vi "CPU Load Benchmark.vi"(8 "error in (no error)":errorcluster, 11 "SV B-M (Host) in":refnum<class "SV B-M (Host).lvclass">) -> (0 "error out":errorcluster, 3 "SV B-M (Host) out":refnum<class "SV B-M (Host).lvclass">)   [LabVIEW 2015, in "SV B-M (Host).lvclass"]
doc: "Open connections to all the shared variables that were deployed. Send a command to the target to do the same and wait for acknowledgement that was completed."
uses:
  SV B-M (Host).lvclass
  SV B-M (Host).lvclass/SV B-M (Host).ctl
  Listbox - In Progress.vi
  Command & Ack - Send Command.vi
  Command & Ack - Receive Ack.vi
  Process Ack Data - CPU Load BM.vi
  Listbox - Complete.vi
panel:
  out "SV Data":variant[][](array[variant])
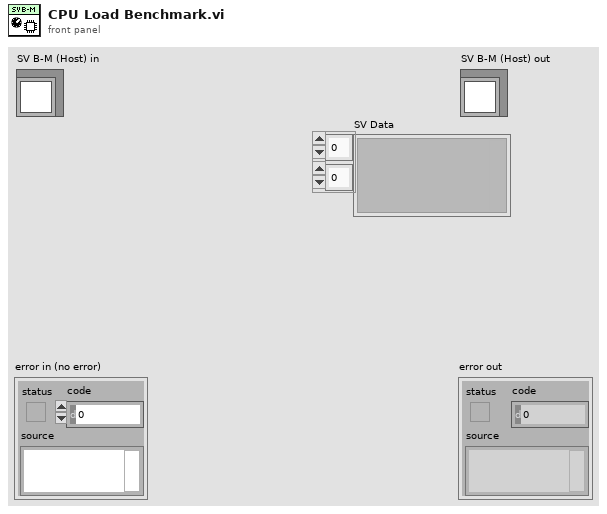
[diagram p1: front panel]
types:
  T1 = typedef "Variable Data Type.ctl" = enum16{"U8", "U16", "U32", "U64", "I8", "I16", "I32", "I64", "Single", "Double", "Boolean", "String"}
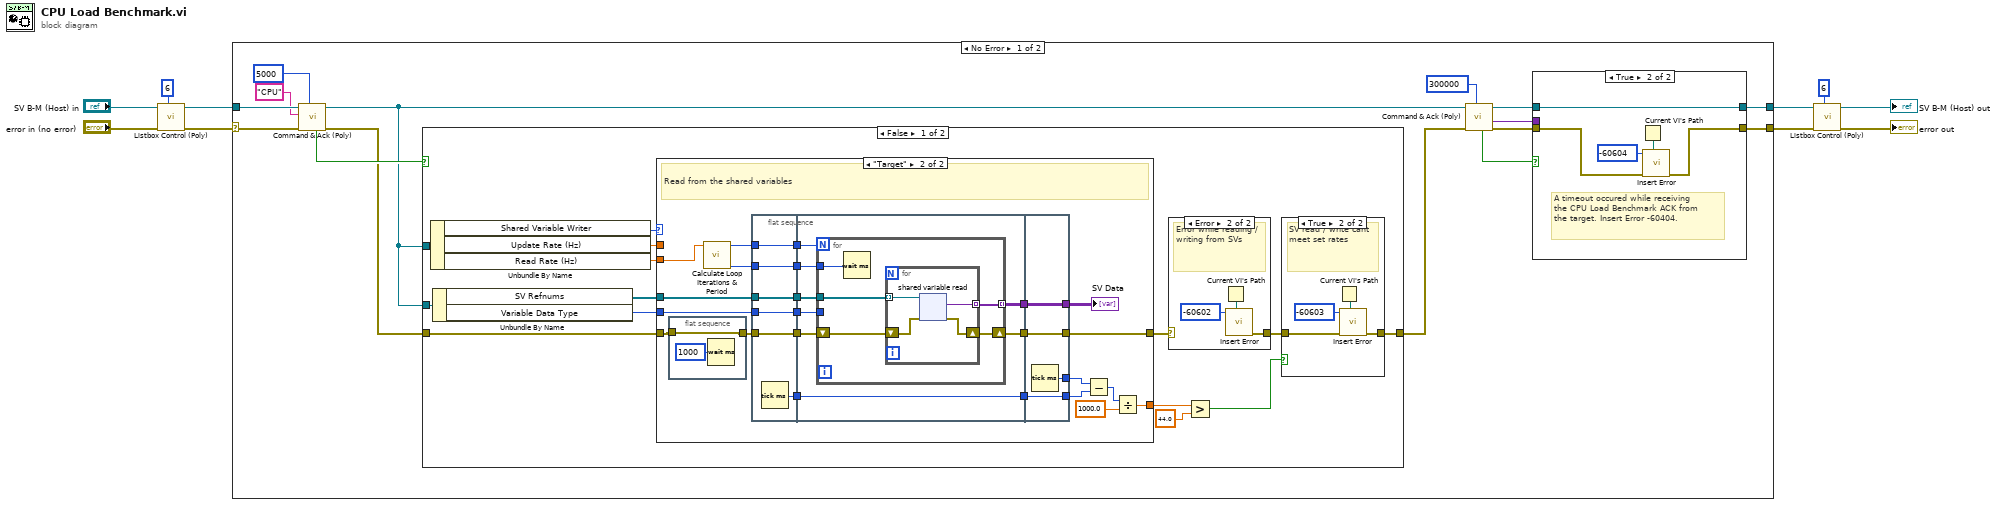
[diagram p0: block diagram]
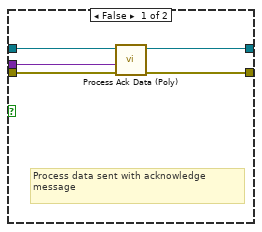
[diagram p2: hidden frame]
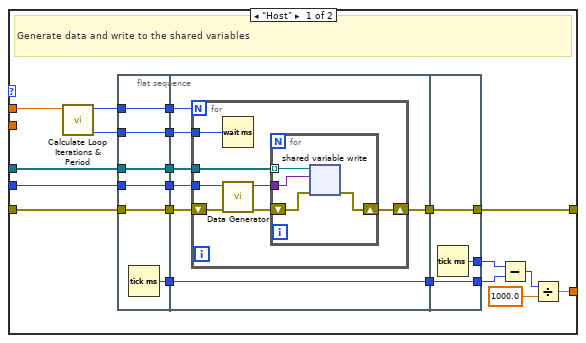
[diagram p5: hidden frame]
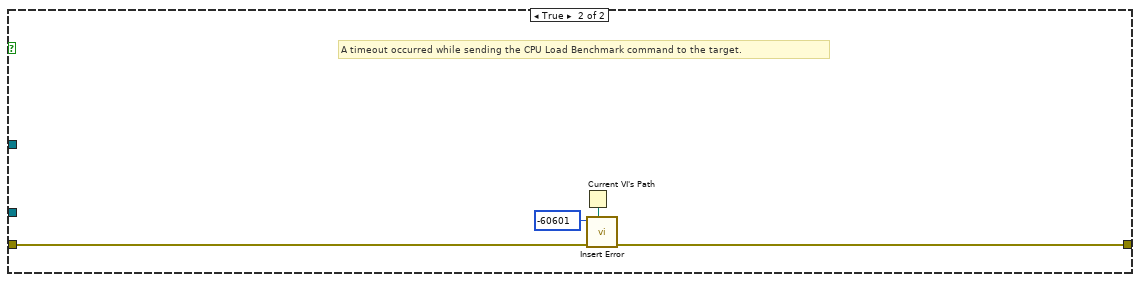
[diagram p6: hidden frame]
diagram:
  n1 = call-poly "Listbox Control (Poly).vi"("Row to Update"=6, "error in (no error)"="error in (no error)", "SV B-M In"="SV B-M (Host) in") -> ("error out"=w7:errorcluster, "SV B-M Out"=w8:refnum<class "SV B-M (Host).lvclass">)  [unwired: 7 in]
  n2 = case shown="No Error" w7 {
    selector: w7 -> [w24 w163]
    tunnel: [w12 w163] -> w3
    tunnel: [w13 w162] -> w4
    tunnel: w8 -> [w25 w162]
    frame No Error {
      n3 = call-poly "Command & Ack (Poly).vi"("Timeout (-1)"=5000, "error in (no error)"=w24, "Message"="CPU", "SV B-M (Host) in"=w25) -> ("error out"=w19:errorcluster, "SV B-M (Host) out"=w18:refnum<class "SV B-M (Host).lvclass">, "Timeout?"=w20:bool)  [unwired: 5 in]
      n4 = case shown="False" w20 {
        tunnel: w19 -> [w42 w161]
        tunnel: w18 -> [w49 _]
        tunnel: w18 -> [w45 _]
        tunnel: [w36 w158] -> w17
        frame False {
          n5 = Unbundle By Name(w49) -> ("Shared Variable Writer"=w48:enum16{"Target", "Host"}, "Update Rate (Hz)"=w47:dbl, "Read Rate (Hz)"=w46:dbl)
          n6 = Unbundle By Name(w45) -> ("SV Refnums"=w44:refnum<k21>[], "Variable Data Type"=w43:T1)
          n7 = case shown="\"Target\"" w48 {
            tunnel: w47 -> [w78 _]
            tunnel: w46 -> [_ w111]
            tunnel: w44 -> [w75 w126]
            tunnel: w43 -> [w74 w125]
            tunnel: w42 -> [w69 w107]
            tunnel: [w60 w112] -> w41
            tunnel: [w59 w109] -> w39
            frame "Host" {
              # "Generate data and write to the shared variables"
              n8 = call "Calculate Loop Iterations & Period.vi"("Rate"=w78) -> ("Wait (ms)"=w76:u32, "# Iterations"=w77:i32)  [unwired: 9 in]
              n9 = flat-sequence {
                tunnel: w74 -> [w81]
                tunnel: w75 -> [w82]
                tunnel: w76 -> [w83]
                tunnel: w77 -> [w84]
                tunnel: [w84] -> w73
                tunnel: [w83] -> w72
                tunnel: [w82] -> w71
                tunnel: [w81] -> w70
                tunnel: w69 -> [w80]
                tunnel: [w80] -> w68
                tunnel: [w79] -> w67
                tunnel: w73 -> [w91]
                tunnel: w72 -> [w90]
                tunnel: w71 -> [w89]
                tunnel: w70 -> [w88]
                tunnel: w68 -> [w87]
                tunnel: w67 -> [w86]
                tunnel: [w86] -> w66
                tunnel: [w85] -> w65
                tunnel: [w105] -> w64
                tunnel: w66 -> [w105]
                tunnel: w65 -> [w103]
                tunnel: [w104] -> w63
                tunnel: [w103] -> w59
                frame #0 {
                  n10 = Tick Count (ms)() -> (millisecond timer value=w79:u32)
                }
                frame #1 {
                  n11 = for {
                    N: w91 -> [_]
                    tunnel: w90 -> [w98]
                    tunnel: w89 -> [w95]
                    tunnel: w88 -> [w97]
                    shift-right: [w92] -> w85
                    shift-left: w87 -> [w96]
                    n12 = Wait (ms)(milliseconds to wait=w98) -> ()  [unwired: 1 out]
                    n13 = call "Data Generator.vi"("error in (no error)"=w96, "Variable Data Type"=w97) -> ("error out"=w93:errorcluster, "Variant"=w94:variant)  [unwired: 8 in]
                    n14 = for {
                      tunnel: w95 -> [w102] mode=indexing
                      tunnel: w94 -> [w100]
                      shift-right: [w99] -> w92
                      shift-left: w93 -> [w101]
                      n15 = shared-variable-write(w102, w101, w100) -> (w99:errorcluster)  [unwired: 1 out]
                    }
                  }
                }
                frame #2 {
                  n16 = Tick Count (ms)() -> (millisecond timer value=w104:u32)
                }
              }
              n17 = Subtract(x=w63, y=w64) -> (x-y=w62:u32)
              n18 = Divide(x=w62, y=1000.0) -> (x/y=w60:dbl)
            }
            frame "Target" {
              # "Read from the shared variables"
              n19 = flat-sequence {
                tunnel: [w130] -> w106
                tunnel: w107 -> [w130]
                frame #0 {
                  n20 = Wait (ms)(milliseconds to wait=u32 1000) -> ()  [unwired: 1 out]
                }
              }
              n21 = call "Calculate Loop Iterations & Period.vi"("Rate"=w111) -> ("Wait (ms)"=w127:u32, "# Iterations"=w128:i32)  [unwired: 9 in]
              n22 = flat-sequence {
                tunnel: w125 -> [w133]
                tunnel: w126 -> [w134]
                tunnel: w127 -> [w135]
                tunnel: w128 -> [w136]
                tunnel: [w136] -> w124
                tunnel: [w135] -> w123
                tunnel: [w134] -> w122
                tunnel: [w133] -> w121
                tunnel: w106 -> [w132]
                tunnel: [w132] -> w120
                tunnel: [w131] -> w119
                tunnel: w124 -> [w144]
                tunnel: w123 -> [w143]
                tunnel: w122 -> [w142]
                tunnel: w121 -> [w141]
                tunnel: w120 -> [w140]
                tunnel: w119 -> [w139]
                tunnel: [w139] -> w118
                tunnel: [w138] -> w117
                tunnel: [w137] -> w110
                tunnel: [w157] -> w116
                tunnel: w118 -> [w157]
                tunnel: w117 -> [w154]
                tunnel: [w156] -> w115
                tunnel: [w155] -> w108
                tunnel: w110 -> [w155]
                tunnel: [w154] -> w109
                frame #0 {
                  n23 = Tick Count (ms)() -> (millisecond timer value=w131:u32)
                }
                frame #1 {
                  n24 = for {
                    N: w144 -> [_]
                    tunnel: w143 -> [w149]
                    tunnel: w142 -> [w148]
                    tunnel: w141 -> [_]
                    shift-right: [w147] -> w138
                    shift-left: w140 -> [w146]
                    tunnel: [w145] -> w137 mode=indexing
                    n25 = Wait (ms)(milliseconds to wait=w149) -> ()  [unwired: 1 out]
                    n26 = for {
                      tunnel: w148 -> [w153] mode=indexing
                      shift-right: [w151] -> w147
                      shift-left: w146 -> [w152]
                      tunnel: [w150] -> w145 mode=indexing
                      n27 = shared-variable-read(w153, w152) -> (w151:errorcluster, w150:variant)  [unwired: 2 out]
                    }
                  }
                }
                frame #2 {
                  n28 = Tick Count (ms)() -> (millisecond timer value=w156:u32)
                }
              }
              n29 = Subtract(x=w115, y=w116) -> (x-y=w114:u32)
              n30 = Divide(x=w114, y=1000.0) -> (x/y=w112:dbl)
              "SV Data" <- w108
            }
          }
          n31 = case shown="Error" w39 {
            selector: w39 -> [w55 _]
            tunnel: [w55 w56] -> w38
            frame No Error {
              # "No Error"
            }
            frame Error {
              # "Error while reading / writing from SVs"
              n32 = Current VI's Path() -> (path=w58:path)
              n33 = call "Insert Error.vi"("VI Path"=w58, "Error Code"=-60602) -> ("error out"=w56:errorcluster)  [unwired: 9 in]
            }
          }
          n34 = Greater?(x=w41, y=44.0) -> (0:w37:bool)
          n35 = case shown="True" w37 {
            tunnel: [w50 w52] -> w36
            tunnel: w38 -> [w50 w51]
            frame False {
              # "R/W rates met\nwithin 10%"
            }
            frame True {
              # "SV read / write cant\nmeet set rates"
              n36 = Current VI's Path() -> (path=w54:path)
              n37 = call "Insert Error.vi"("VI Path"=w54, "error in (no error)"=w51, "Error Code"=-60603) -> ("error out"=w52:errorcluster)  [unwired: 8 in]
            }
          }
        }
        frame True {
          # "A timeout occurred while sending the CPU Load Benchmark command to the target."
          n38 = Current VI's Path() -> (path=w159:path)
          n39 = call "Insert Error.vi"("VI Path"=w159, "error in (no error)"=w161, "Error Code"=-60601) -> ("error out"=w158:errorcluster)  [unwired: 8 in]
        }
      }
      n40 = call-poly "Command & Ack (Poly).vi"("Timeout (-1)"=300000, "error in (no error)"=w17, "SV B-M (Host) in"=w18) -> ("error out"=w15:errorcluster, "Message Data"=w11:variant, "SV B-M (Host) out"=w16:refnum<class "SV B-M (Host).lvclass">, "Timeout?"=w14:bool)  [unwired: 4 in, 1 out]
      n41 = case shown="True" w14 {
        tunnel: w16 -> [w30 w35]
        tunnel: w15 -> [w28 w34]
        tunnel: [w27 w35] -> w13
        tunnel: [w26 w31] -> w12
        tunnel: w11 -> [w29 _]
        frame False {
          # "Process data sent with acknowledge\nmessage"
          n42 = call-poly "Process Ack Data (Poly).vi"("error in (no error)"=w28, "CPU Load Data"=w29, "SV B-M (Host) in"=w30) -> ("error out"=w26:errorcluster, "SV B-M (Host) out"=w27:refnum<class "SV B-M (Host).lvclass">)  [unwired: 7 in]
        }
        frame True {
          # "A timeout occured while receiving\nthe CPU Load Benchmark ACK from\nthe target. Insert Error -60404."
          n43 = Current VI's Path() -> (path=w32:path)
          n44 = call "Insert Error.vi"("VI Path"=w32, "error in (no error)"=w34, "Error Code"=-60604) -> ("error out"=w31:errorcluster)  [unwired: 8 in]
        }
      }
    }
    frame Error {
    }
  }
  n45 = call-poly "Listbox Control (Poly).vi"("Row to Update"=6, "error in (no error)"=w3, "SV B-M In"=w4) -> ("error out"=→"error out":errorcluster, "SV B-M Out"=→"SV B-M (Host) out":refnum<class "SV B-M (Host).lvclass">)  [unwired: 7 in]
